vi "Actor Core.vi"(8 "error in":errorcluster, 11 "Nested in":refnum<class "Normal Log.lvclass">) -> (0 "error out":errorcluster, 3 "Actor out":refnum<class "Actor.lvclass">)   [LabVIEW 2020, in "Normal Log.lvlib" / "Normal Log.lvclass"]
doc: "(<B>Filename</B>: Actor Framework.lvlib:Actor.lvclass:Actor Core.vi)\n\nReceives messages to the actor, reacts to them, and initiates any error handling that may shut the actor down.\n\nDescendant classes may override this VI to append parallel tasks for the actor to complete while it handles messages. Overrides use the Call Parent Method node."
uses:
  Normal Log.lvclass
  <vilib>/ActorFramework/Actor/Actor.lvclass
  <vilib>/ActorFramework/Stop Msg/Stop Msg.lvclass
  Log/Log/Log.lvclass
  Normal Log Messages/Event Adaptive Size Msg/Event Adaptive Size Msg.lvclass
panel:
  in  "log":i32(listbox)
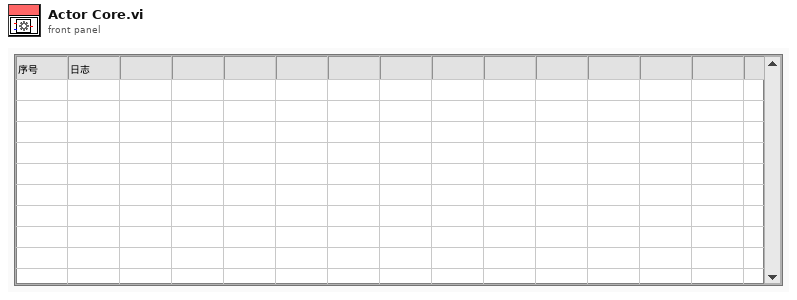
[diagram p1: front panel]
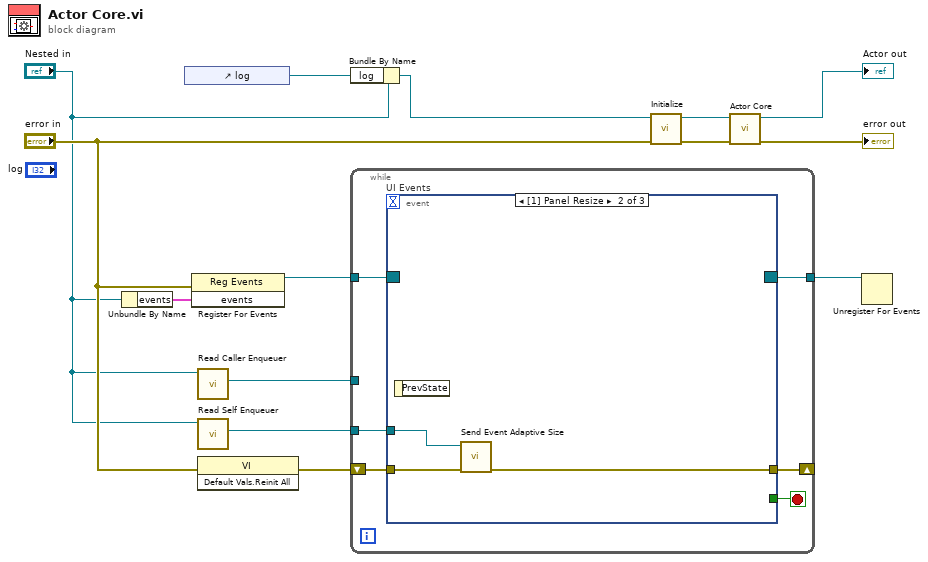
[diagram p0: block diagram]
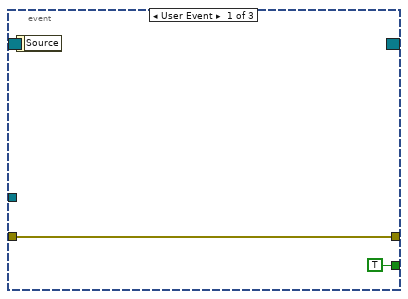
[diagram p2: hidden frame]
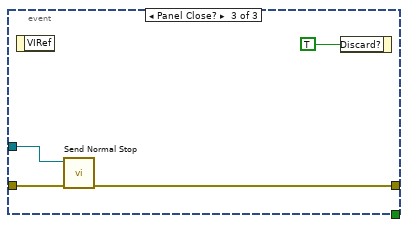
[diagram p3: hidden frame]
diagram:
  n1 = Unbundle By Name("Nested in") -> ("events"=w11:cluster{"stop":refnum<user-event>})
  n2 = control-ref of="log"() -> (w2:refnum<vi>)
  n3 = register-events ("Main Register for Events")(error in="error in", w11) -> (reference out=w12:refnum<event-registration>)  [unwired: 1 in, 1 out]
  n4 = call <vilib>:"Read Caller Enqueuer.vi"("Actor"="Nested in") -> ("Caller Enqueuer"=w8:refnum<class "Message Enqueuer.lvclass">)  [unwired: 10 in]
  n5 = call <vilib>:"Read Self Enqueuer.vi"("Actor"="Nested in") -> ("Self Enqueuer"=w9:refnum<class "Message Enqueuer.lvclass">)  [unwired: 10 in]
  n6 = invoke class="VI" method="Default Vals.Reinit All"(error in="error in") -> (error out=w7:errorcluster)  [unwired: 2 in, 2 out]
  n7 = Bundle By Name(cluster="Nested in", "log"=w2) -> (w1:refnum<class "Normal Log.lvclass">)
  n8 = while {
    tunnel: w12 -> [w20]
    tunnel: [w18] -> w10
    tunnel: w9 -> [w17]
    tunnel: w8 -> [_]
    shift-right: [w15] -> _
    shift-left: w7 -> [w16]
    stop <- w19 stop-if-true
    n9 = event "UI Events" shown="[1] Panel Resize" {
      selector: w20 -> [_ _ _]
      dyn-events: [_ _ _] -> w18
      timeout: _ -> [_ _ _]
      tunnel: [TRUE _ _] -> w19
      tunnel: w17 -> [_ w24 w28]
      tunnel: w16 -> [w22 w25 w27]
      tunnel: [w22 w23 w26] -> w15
      event User Event {
        n10 = event-data() -> ()  [unwired: 1 in, 1 out]
      }
      event Panel Resize {
        n11 = event-data() -> ()  [unwired: 1 in, 1 out]
        n12 = call "Send Event Adaptive Size.vi"("error in (no error)"=w25, "Message Enqueuer"=w24) -> ("error out"=w23:errorcluster)  [unwired: 8 in, 1 out]
      }
      event Panel Close? {
        n13 = event-data() -> ()  [unwired: 1 in, 1 out]
        n14 = call <vilib>:"Send Normal Stop.vi"("error in (no error)"=w27, "Message Enqueuer"=w28) -> ("error out"=w26:errorcluster)  [unwired: 9 in]
        n15 = event-data("Discard?"=TRUE) -> ()  [unwired: 1 in, 1 out]
      }
    }
  }
  n16 = call "Initialize.vi"("error in (no error)"="error in", "View Template in"=w1) -> ("error out"=w6:errorcluster, "View Template out"=w5:refnum<class "Normal Log.lvclass">)  [unwired: 8 in]
  n17 = call-parent "Actor Core.vi"("error in"=w6, "Log in"=w5) -> ("error out"=→"error out":errorcluster, "Actor out"=→"Actor out":refnum<class "Actor.lvclass">)  [unwired: 8 in]
  n18 = Unregister For Events(event registration refnum=w10) -> ()  [unwired: 1 in, 1 out]
